vi "Brent with Derivatives 1D.vi"(4 "accuracy":dbl=1e-08 format="%.0e", 5 "formula":string, 6 "c (start)":dbl format="%.2f", 7 "b (start)":dbl format="%.2f", 8 "a (start)":dbl format="%.2f") -> (0 "error":i32, 1 "ticks":u32, 2 "f(minimum)":dbl format="%.2f", 3 "minimum":dbl format="%.2f")   [LabVIEW 2014, in "NI_Gmath.lvlib"]
doc: "Determines a local minimum of a given 1D function in a given interval. The method is based on derivatives of the function."
uses:
  NI_Gmath.lvlib
panel:
  # "Example:\n\n accuracy: 1E-8 \n a (start): 0.0 \n b (start): 0.5\n c (start): 1.0 \n formula: (x-(3/10))^2+1"
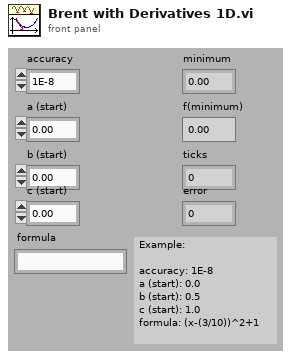
[diagram p1: front panel]
types:
  T1 = cluster{"c (start)":dbl, "c (start)":dbl, "c (start)":dbl}
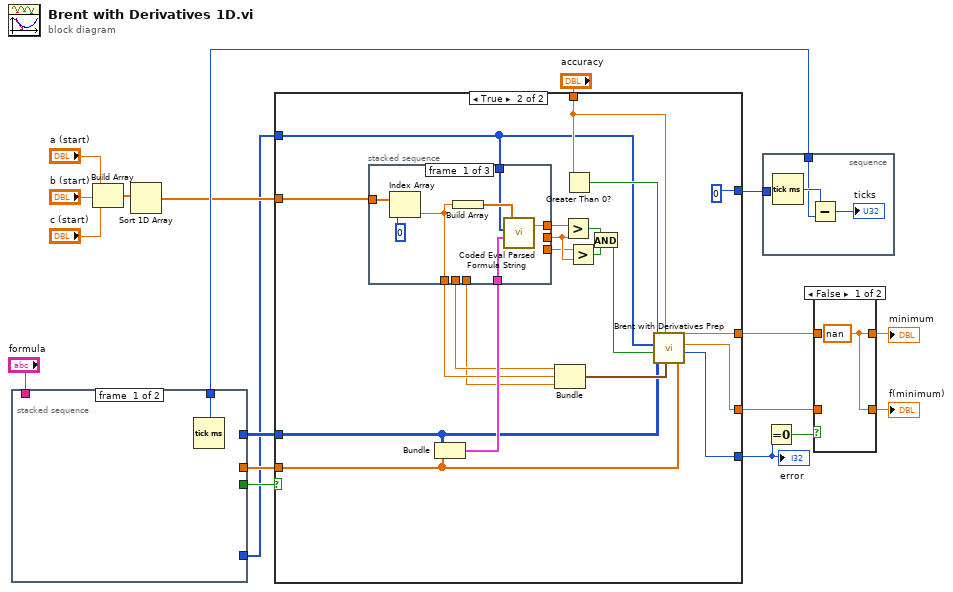
[diagram p0: block diagram]
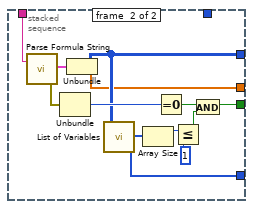
[diagram p3: hidden frame]
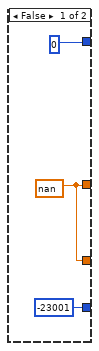
[diagram p4: hidden frame]
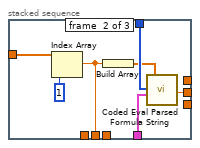
[diagram p5: hidden frame]
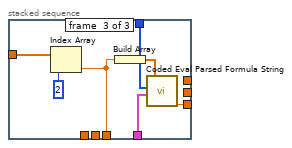
[diagram p6: hidden frame]
diagram:
  n1 = stacked-sequence {
    tunnel: [_ w32] -> w18
    tunnel: [w20 _] -> w17
    tunnel: "formula" -> [_ w26]
    tunnel: [_ w22] -> w3
    tunnel: [_ w21] -> w2
    tunnel: [_ w27] -> w1
    frame #0 {
      n2 = Tick Count (ms)() -> (millisecond timer value=w20:u32)
    }
    frame #1 {
      n3 = call "Parse Formula String.vi"("formula"=w26) -> ("error out"=w25:errorcluster, "Parsed Formula"=w23:cluster{"Table":i32[][], "Y Values":dbl[]})  [unwired: 1 in]
      n4 = Unbundle(w25) -> ("code"=w24:i32)  [unwired: 2 out]
      n5 = Unbundle(w23) -> ("Table"=w22:i32[][], "Y Values"=w21:dbl[])
      n6 = call "List of Variables.vi"("Table"=w22) -> ("List of variables"=w27:i32[])
      n7 = Array Size(array=w27) -> (size(s)=w28:i32)
      n8 = Equal To 0?(x=w24) -> (x = 0?=w31:bool)
      n9 = Less Or Equal?(x=w28, y=1) -> (x <= y?=w30:bool)
      n10 = And(x=w31, y=w30) -> (x .and. y?=w32:bool)
    }
  }
  n11 = Build Array("a (start)", "b (start)", "c (start)") -> (w13:dbl[])
  n12 = Sort 1D Array(array=w13) -> (sorted array=w12:dbl[])
  n13 = case shown="True" w18 {
    tunnel: [0 0] -> w19
    tunnel: w12 -> [_ w55]
    tunnel: [w34 w48] -> w8
    tunnel: [w34 w47] -> w6
    tunnel: [-23001 w45] -> w10
    tunnel: "accuracy" -> [_ w39]
    tunnel: w3 -> [_ w38]
    tunnel: w2 -> [_ w37]
    tunnel: w1 -> [_ w36]
    frame False {
      w34 = nan
    }
    frame True {
      n14 = Bundle("Table"=w38, "Y Values"=w37) -> (w44:cluster{"Table":i32[][], "Y Values":dbl[]})  [unwired: 1 in]
      n15 = stacked-sequence {
        tunnel: w55 -> [w63 w70 w77]
        tunnel: w36 -> [w58 w66 w72]
        tunnel: [w61 _ _] -> w54
        tunnel: [_ w68 _] -> w53
        tunnel: [_ _ w75] -> w52
        tunnel: [w60 _ _] -> w42
        tunnel: [_ w67 _] -> w43
        tunnel: [_ _ w74] -> w41
        tunnel: w44 -> [w57 w64 w71]
        frame #0 {
          n16 = Index Array(array=w63, index=0) -> (element=w60:dbl)
          n17 = Build Array(w60) -> (w59:dbl[])
          n18 = call "Coded Eval Parsed Formula String.vi"("Parsed Formula"=w57, "Variables"=w58, "X Values"=w59) -> ("y value"=w61:dbl)  [unwired: 1 in, 1 out]
        }
        frame #1 {
          n19 = Index Array(array=w70, index=1) -> (element=w67:dbl)
          n20 = Build Array(w67) -> (w65:dbl[])
          n21 = call "Coded Eval Parsed Formula String.vi"("Parsed Formula"=w64, "Variables"=w66, "X Values"=w65) -> ("y value"=w68:dbl)  [unwired: 1 in, 1 out]
        }
        frame #2 {
          n22 = Index Array(array=w77, index=2) -> (element=w74:dbl)
          n23 = Build Array(w74) -> (w73:dbl[])
          n24 = call "Coded Eval Parsed Formula String.vi"("Parsed Formula"=w71, "Variables"=w72, "X Values"=w73) -> ("y value"=w75:dbl)  [unwired: 1 in, 1 out]
        }
      }
      n25 = Bundle("c (start)"=w43, "c (start)"=w42, "c (start)"=w41) -> (w40:T1)  [unwired: 1 in]
      n26 = Greater?(x=w54, y=w53) -> (0:w51:bool)
      n27 = Greater Than 0?(x=w39) -> (x > 0?=w46:bool)
      n28 = Greater?(x=w52, y=w53) -> (0:w50:bool)
      n29 = And(x=w51, y=w50) -> (x .and. y?=w49:bool)
      n30 = call "Brent with Derivatives Prep.vi"("result"=w37, "values"=w40, "accuracy"=w39, "table"=w38, "inner case"=w49, "list of variables"=w36, "outer case"=w46) -> ("error"=w45:i32, "f(minimum)"=w47:dbl, "minimum"=w48:dbl)
    }
  }
  "error" <- w10
  n31 = stacked-sequence {
    tunnel: w17 -> [w79]
    tunnel: w19 -> [_]
    frame #0 {
      n32 = Tick Count (ms)() -> (millisecond timer value=w80:u32)
      n33 = Subtract(x=w80, y=w79) -> (x-y=→"ticks":u32)
    }
  }
  n34 = Equal To 0?(x=w10) -> (x = 0?=w9:bool)
  n35 = case shown="False" w9 {
    tunnel: w8 -> [_ w83]
    tunnel: [w81 w83] -> w7
    tunnel: w6 -> [_ w82]
    tunnel: [w81 w82] -> w5
    frame False {
      w81 = nan
    }
    frame True {
    }
  }
  "minimum" <- w7
  "f(minimum)" <- w5
